vi "_XNET Convert Time LV to U64 100ns.vi"(3 "Time LV":timestamp) -> (1 "Time U64 100ns":u64)   [LabVIEW 2018]
uses:
  nixlvapi.dll
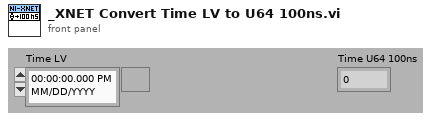
[diagram p1: front panel]
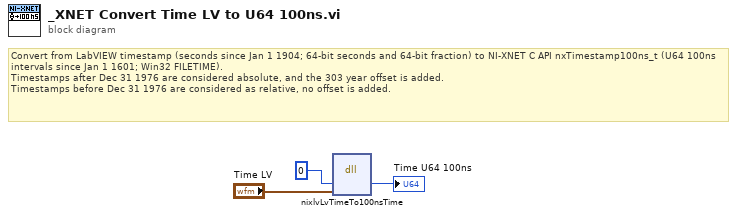
[diagram p0: block diagram]
diagram:
  # "Convert from LabVIEW timestamp (seconds since Jan 1 1904; 64-bit seconds and 64-bit fraction) to NI-XNET C API nxTimestamp100ns_t (U64 100ns intervals since Jan 1 1601; Win32 FILETIME).\nTimestamps after Dec 31 1976 are considered absolute, and the 303 year offset is added.\nTimestamps before Dec 31 1976 are considered as relative, no offset is added."
  n1 = dll-call lib="nixlvapi.*" fn="nixlvLvTimeTo100nsTime" label="Call Library"("cTime"=u64 0 ("rawTime"), "lvTime"="Time LV") -> ("cTime"=→"Time U64 100ns":u64)  [unwired: 4 in, 3 out]
